vi "Serial Write.vi"(8 "error in (no error)":errorcluster, 9 "Serial Settings":T1={"baud rate"=115200, "data bits"=8, "parity"=enum."None", "stop bits"=10, "flow control"=0} {"flow control" items=["None"=0, "XON/XOFF"=1, "RTS/CTS"=2, "DTR/DSR"=4]; "stop bits" items=["1.0"=10, "1.5"=15, "2.0"=20]; "data bits" min=5 max=8 step=1; "baud rate" items=["75"=75, "110"=110, "134"=134, "150"=150, "300"=300, "600"=600, "1200"=1200, "1800"=1800, "2400"=2400, "4800"=4800, "7200"=7200, "9600"=9600, "14400"=14400, "19200"=19200, "28800"=28800, "38400"=38400, "56000"=56000, "57600"=57600, "115200"=115200, "128000"=128000, "230400"=230400]}, 10 "Command":string, 11 "VISA resource name":refnum<visa-resource-name>="COM1") -> (0 "error out":errorcluster, 1 "Pass?":bool, 2 "bytes read":u32, 3 "Response":string)   [LabVIEW 2025]
doc: "This example performs a serial port write and a serial port read. The parameters set for the serial port must match the parameters of the connected instrument or device. The VISA Configure Serial Port VI sets the configuration parameters. The front panel displays the controls used to configure the basic parameters, such as baud rate, data bits, and parity. The VI passes the VISA resource name to other VIs that perform operations on that VISA resource. The VISA Write function sends a command to the serial device and the VISA Read function returns data based on the command. The VISA Close function then closes the reference to the serial device. It is important to close the reference; otherwise, further communication through that port might not be possible."
uses:
  Program Files (x86)/National Instruments/LabVIEW 2025/examples/Instrument IO/Serial/support/Serial - Settings.ctl
  <vilib>/Instr/_visa.llb/VISA Configure Serial Port (Instr).vi
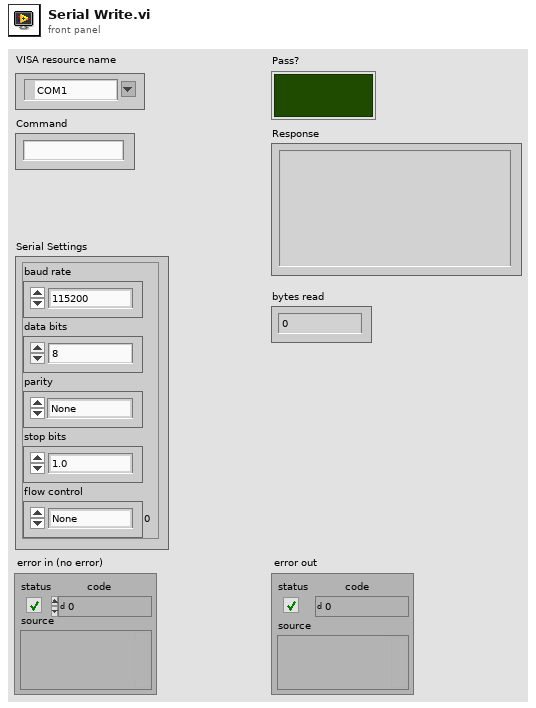
[diagram p1: front panel]
types:
  T1 = typedef "Serial - Settings.ctl" = cluster{"baud rate":u32, "data bits":u16, "parity":enum16{"None", "Odd", "Even", "Mark", "Space"}, "stop bits":u16, "flow control":u16}
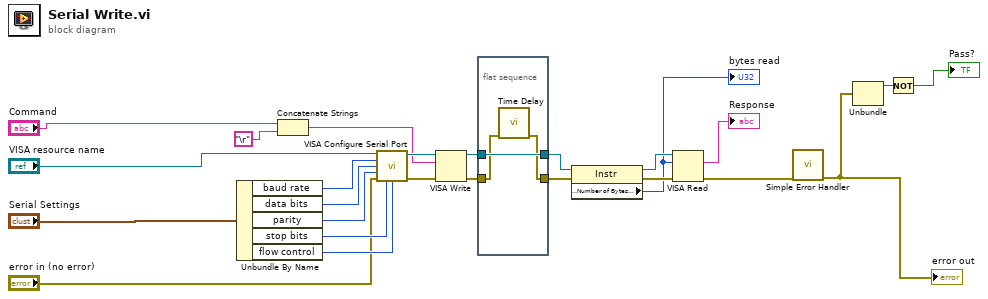
[diagram p0: block diagram]
diagram:
  n1 = Unbundle By Name("Serial Settings") -> ("baud rate"=w14:u32, "data bits"=w13:u16, "parity"=w12:enum16{"None", "Odd", "Even", "Mark", "Space"}, "stop bits"=w11:u16, "flow control"=w10:u16)
  n2 = Concatenate Strings("Command", "\r") -> (w9:string)
  n3 = call-poly "VISA Configure Serial Port"("VISA resource name"="VISA resource name", "baud rate (9600)"=w14, "data bits (8)"=w13, "parity (0:none)"=w12, "error in (no error)"="error in (no error)", "stop bits (10: 1 bit)"=w11, "flow control (0:none)"=w10) -> ("VISA resource name out"=w23:refnum<visa-resource-name>, "error out"=w24:errorcluster)  [unwired: 2 in, 5 out]
  n4 = VISA Write(VISA resource name=w23, write buffer=w9, error in (no error)=w24) -> (VISA resource name out=w21:refnum<visa-resource-name>, error out=w2:errorcluster)  [unwired: 1 out]
  n5 = flat-sequence {
    tunnel: w21 -> [w28]
    tunnel: [w28] -> w20
    tunnel: w2 -> [w27]
    tunnel: [w26] -> w1
    frame #0 {
      n6 = call "Time Delay"("error in (no error)"=w27) -> ("error out"=w26:errorcluster)  [unwired: 10 in]
    }
  }
  n7 = property class="Instr"(reference=w20, error in=w1) -> (reference out=w19:refnum<visa-resource-name>, error out=w18:errorcluster, "Serial Settings:Number of Bytes at Serial Port"=w16:u32)
  "bytes read" <- w16
  n8 = VISA Read(VISA resource name=w19, byte count=w16, error in (no error)=w18) -> (read buffer=→"Response":string, error out=w22:errorcluster)  [unwired: 2 out]
  n9 = call <vilib>:"Simple Error Handler.vi"("error in (no error)"=w22) -> ("error out"=w5:errorcluster)  [unwired: 1 in, 7 out]
  "error out" <- w5
  n10 = Unbundle(w5) -> ("status"=w4:bool)  [unwired: 2 out]
  n11 = Not(x=w4) -> (.not. x?=→"Pass?":bool)
